vi "RT Loop - Acquire camera.vi"(11 "Camera Queue  in":refnum<k33>) -> (0 "error out":errorcluster)   [LabVIEW 2017]
uses:
  <vilib>/vision/Image Controls.llb/IMAQ Image.ctl
  UI Error Handlers/support/Message Queue/Message Cluster.ctl
  <vilib>/userdefined/High Color/IMAQdx.ctl
  Globals/Global - All RT Loop Stop.vi
  <vilib>/vision/driver/NI_Vision_Acquisition_Software.lvlib
  UI Error Handlers/support/Message Queue/Message Queue.lvlib
panel:
  in  "Message Queue":refnum<queue>
  in  "G1 Trigger":bool=TRUE
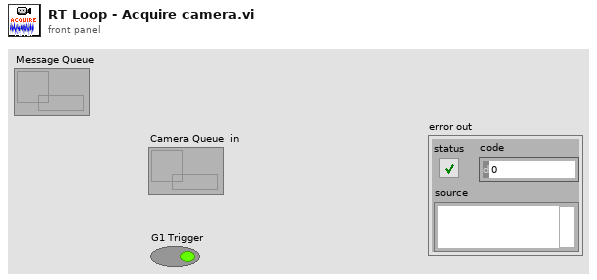
[diagram p1: front panel]
types:
  T1 = typedef "IMAQ Image.ctl" = refnum<image>
  T2 = typedef "IMAQdx.ctl" = refnum<k21>
  T3 = typedef "Image Type" = u32
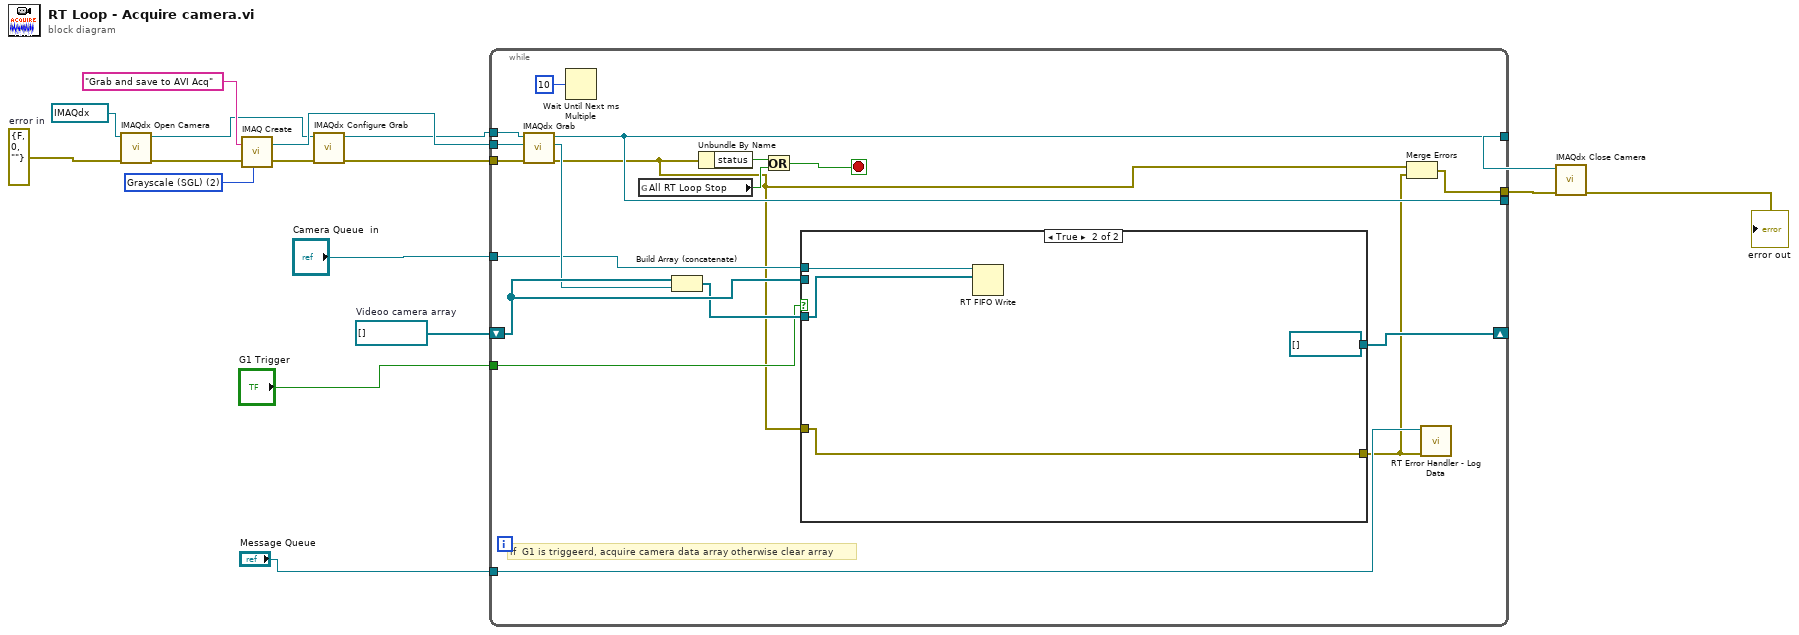
[diagram p0: block diagram]
diagram:
  w15 = T1[] []  # Videoo camera array
  w8 = T3 2 items=["Grayscale (U8)", "Grayscale (I16)", "Grayscale (SGL)", "Complex (CSG)", "RGB (U32)", "HSL (U32)", "RGB (U64)", "Grayscale (U16)"] ("Image Type")
  w6 = errorcluster {"status"=FALSE, "code"=0, "source"=""}  # error in
  n1 = call <vilib>:"IMAQdx Open Camera.vi"("error in"=w6, "Session In"=T2 "cam0") -> ("error out"=w9:errorcluster, "Session Out"=w4:T2)  [unwired: 8 in]
  n2 = call "IMAQ Create"("Image Name"="Grab and save to AVI Acq", "Image Type"=w8, "error in (no error)"=w9) -> ("New Image"=w12:T1, "error out"=w13:errorcluster)  [unwired: 2 in]
  n3 = call <vilib>:"IMAQdx Configure Grab.vi"("error in"=w13, "Session In"=w4) -> ("error out"=w14:errorcluster, "Session Out"=w11:T2)  [unwired: 8 in]
  n4 = while {
    tunnel: [w25] -> _
    shift-right: [w22] -> _
    shift-left: w15 -> [w32]
    tunnel: "Camera Queue  in" -> [w30]
    tunnel: w11 -> [w29]
    tunnel: w12 -> [w28]
    tunnel: w14 -> [w27]
    tunnel: [w25] -> w16
    tunnel: "G1 Trigger" -> [w23]
    tunnel: "Message Queue" -> [w21]
    tunnel: [w18] -> w1
    stop <- w26 stop-if-true
    # "if  G1 is triggeerd, acquire camera data array otherwise clear array"
    n5 = call <vilib>:"IMAQdx Grab.vi"("error in"=w27, "Image In"=w28, "Session In"=w29) -> ("error out"=w19:errorcluster, "Image Out"=w31:T1, "Session Out"=w25:T2)  [unwired: 5 in, 1 out]
    n6 = Wait Until Next ms Multiple(millisecond multiple=u32 10 ("milliseconds to wait")) -> ()  [unwired: 1 out]
    n7 = global read "Global - All RT Loop Stop.vi" "All RT Loop Stop"() -> (w33:bool)
    n8 = Build Array (concatenate)(w32, w31) -> (w24:T1[])
    n9 = Unbundle By Name(w19) -> ("status"=w34:bool)
    n10 = Or(x=w34, y=w33) -> (x .or. y?=w26:bool)
    n11 = case shown="True" w23 {
      tunnel: w32 -> [_ _]
      tunnel: [w37 T1[] []] -> w22
      tunnel: w30 -> [_ w41]
      tunnel: w24 -> [w37 w40]
      tunnel: w19 -> [w36 w38]
      tunnel: [w36 w38] -> w20
      frame False {
      }
      frame True {
        n12 = RT FIFO Write(0:w41, 1:w40) -> ()  [unwired: 3 in, 4 out]
      }
    }
    n13 = Merge Errors(w19, w20) -> (w18:errorcluster)
    n14 = call "RT Error Handler - Log Data.vi"("error in (no error)"=w20, "Message Queue"=w21) -> ()  [unwired: 9 in, 1 out]
  }
  n15 = call <vilib>:"IMAQdx Close Camera.vi"("error in"=w1, "Session In"=w16) -> ("error out"=→"error out":errorcluster)  [unwired: 9 in]
